vi "Servo.vi"(8 "error in (no error)":errorcluster, 10 "Servo":dbl min=0.0 max=255.0 step=1.0, 11 "PWM in":refnum<class "PWM.lvclass">) -> (0 "error out":errorcluster, 3 "PWM out":refnum<class "PWM.lvclass">, 5 "data.pwm14":sgl)   [LabVIEW 2020]
uses:
  <vilib>/High Genius/HG_WSI_Tookit/Dependencies/Library/PWM/PWM.lvclass
  C:/Program Files (x86)/National Instruments/LabVIEW 2020/vi.lib/High Genius/HG_WSI_Tookit/Dependencies/Library/HG_LIB/HG_LIB.lvclass
  <vilib>/High Genius/HG_WSI_Tookit/Dependencies/Library/HG_LIB/HG_LIB.lvclass/HG_LIB.ctl
  <vilib>/High Genius/HG_WSI_Tookit/Dependencies/Library/HG_LIB/HG_LIB.lvclass
  <vilib>/High Genius/HG_WSI_Tookit/Dependencies/Library/VMX Library.lvlib
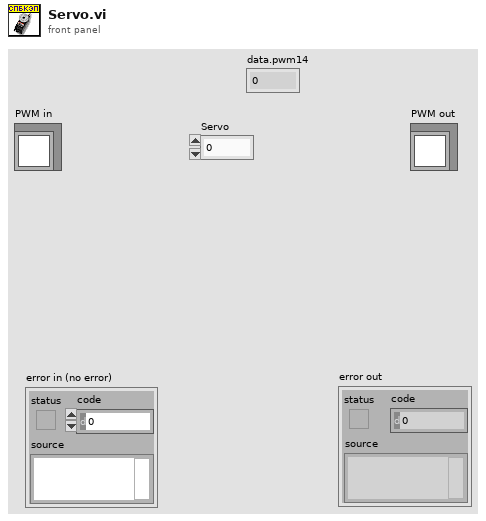
[diagram p1: front panel]
types:
  T1 = typedef "Semaphore RefNum" = refnum<k1>
  T2 = cluster{"titanenc0":i32, "titanenc1":i32, "titanenc2":i32, "titanenc3":i32, "rpm0":i16, "rpm1":i16, "rpm2":i16, "rpm3":i16, "resetenc0":bool, "resetenc1":bool, "resetenc2":bool, "resetenc3":bool}
  T3 = cluster{"data":cluster{"ai22":sgl, "ai23":sgl, "ai24":sgl, "ai25":sgl, "pulse12":i32, "pulse13":i32, "pwm14":i32, "pwm15":i32, "pwm16":dbl, "do17":bool, "do18":bool, "do19":bool, "do20":bool, "do21":bool, "di11":bool, "di9":bool, "motor0":u8, "motor1":u8, "motor2":u8, "motor3":u8, "dir00":u8, "dir01":u8, "dir02":u8, "dir03":u8, "dir10":u8, "dir11":u8, "dir12":u8, "dir13":u8, "limit0":bool, "limit1":bool, "limit2":bool, "limit3":bool, "limit4":bool, "limit5":bool, "limit6":bool, "limit7":bool, "lsb0H":u8, "lsb1H":u8, "lsb2H":u8, "lsb3H":u8, "lsb0L":u8, "lsb1L":u8, "lsb2L":u8, "lsb3L":u8, "enc0_counters":u32, "enc1_counters":u32, "enc2_counters":u32, "enc3_counters":u32, "counter10":u32, "counter8":u32, "reset_enc0":bool, "reset_enc1":bool, "reset_enc2":bool, "reset_enc3":bool, "pitch":sgl, "roll":sgl, "yaw":sgl, "zero_yaw":bool}}
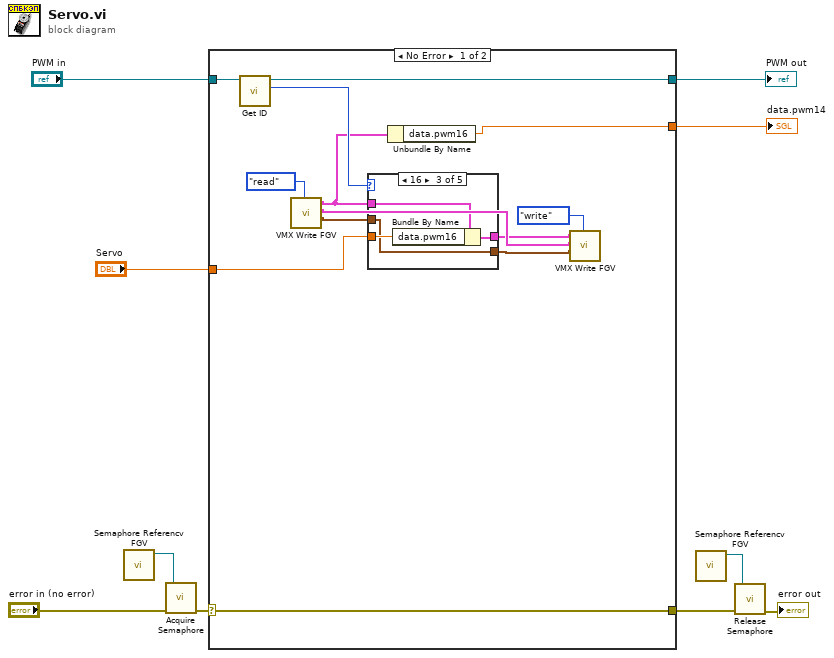
[diagram p0: block diagram]
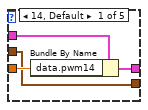
[diagram p2: hidden frame]
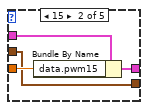
[diagram p3: hidden frame]
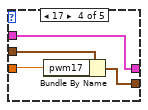
[diagram p4: hidden frame]
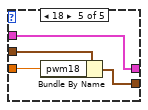
[diagram p5: hidden frame]
diagram:
  n1 = call <vilib>:"Semaphore Referencv FGV.vi"() -> ("Semaphore Reference"=w8:T1)  [unwired: 11 in]
  n2 = call <vilib>:"Acquire Semaphore.vi"("error in (no error)"="error in (no error)", "semaphore"=w8) -> ("error out"=w10:errorcluster)  [unwired: 3 in, 2 out]
  n3 = case shown="No Error" w10 {
    selector: w10 -> [w23 w45]
    tunnel: [w23 w45] -> w6
    tunnel: "PWM in" -> [w22 w44]
    tunnel: [w21 w44] -> w4
    tunnel: "Servo" -> [w19 _]
    tunnel: [w11 _] -> w1
    frame No Error {
      n4 = call <vilib>:"Get ID.vi"("HG_LIB in"=w22) -> ("ID"=w20:u32, "HG_LIB out"=w21:refnum<class "PWM.lvclass">)  [unwired: 9 in]
      n5 = call <vilib>:"VMX Write FGV.vi"("Enum"=enum16{"read", "write"}."read") -> ("Read Data3"=w18:cluster{"pwm17":i32, "pwm18":i32}, "Read Data2"=w17:T2, "Read Data"=w12:T3)  [unwired: 8 in]
      n6 = case shown="16" w20 {
        tunnel: [w27 w30 w32 w38 w42] -> w16
        tunnel: w19 -> [w26 w31 w35 w39 w43]
        tunnel: w12 -> [w25 w28 w34 w38 w42]
        tunnel: w18 -> [w24 w29 w33 w37 w40]
        tunnel: [w24 w29 w33 w36 w41] -> w15
        frame 14, Default {
          n7 = Bundle By Name(cluster=w25, "data.pwm14"=w26) -> (w27:T3)
        }
        frame 15 {
          n8 = Bundle By Name(cluster=w28, "data.pwm15"=w31) -> (w30:T3)
        }
        frame 16 {
          n9 = Bundle By Name(cluster=w34, "data.pwm16"=w35) -> (w32:T3)
        }
        frame 17 {
          n10 = Bundle By Name(cluster=w37, "pwm17"=w39) -> (w36:cluster{"pwm17":i32, "pwm18":i32})
        }
        frame 18 {
          n11 = Bundle By Name(cluster=w40, "pwm18"=w43) -> (w41:cluster{"pwm17":i32, "pwm18":i32})
        }
      }
      n12 = Unbundle By Name(w12) -> ("data.pwm16"=w11:dbl)
      n13 = call <vilib>:"VMX Write FGV.vi"("Enum"=enum16{"read", "write"}."write", "Write Data3"=w15, "Write Data2"=w17, "Write Data"=w16) -> ()  [unwired: 5 in, 3 out]
    }
    frame Error {
    }
  }
  "PWM out" <- w4
  "data.pwm14" <- w1
  n14 = call <vilib>:"Semaphore Referencv FGV.vi"() -> ("Semaphore Reference"=w7:T1)  [unwired: 11 in]
  n15 = call <vilib>:"Release Semaphore.vi"("error in (no error)"=w6, "semaphore"=w7) -> ("error out"=→"error out":errorcluster)  [unwired: 4 in, 1 out]
